vi "testChangeImageBrightness.vi"() -> ()   [LabVIEW 2011, in "run.lvlib"]
uses:
  run.lvlib
  <vilib>/vision/NI_Vision_Development_Module.lvlib
panel:
  out "Maximal Value":sgl
  out "Image Information String":string
  out "Image":T1(plugin-control)
  out "element 2":u32
  in  "stop":bool
  in  "max":dbl(slide) scale=0.0..1604.0
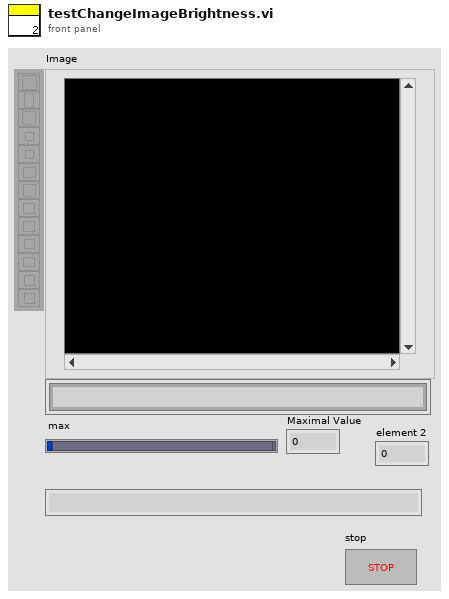
[diagram p1: front panel]
types:
  T1 = typedef "IMAQ Image.ctl" = refnum<image>
  T2 = typedef "Image Type" = u32
  T3 = cluster{"histogram":u32[], "Minimal Value":sgl, "Maximal Value":sgl, "Starting Value":sgl, "Interval Width":sgl, "Mean Value":sgl, "Standard  Variation":sgl, "Area (pixels)":i32}
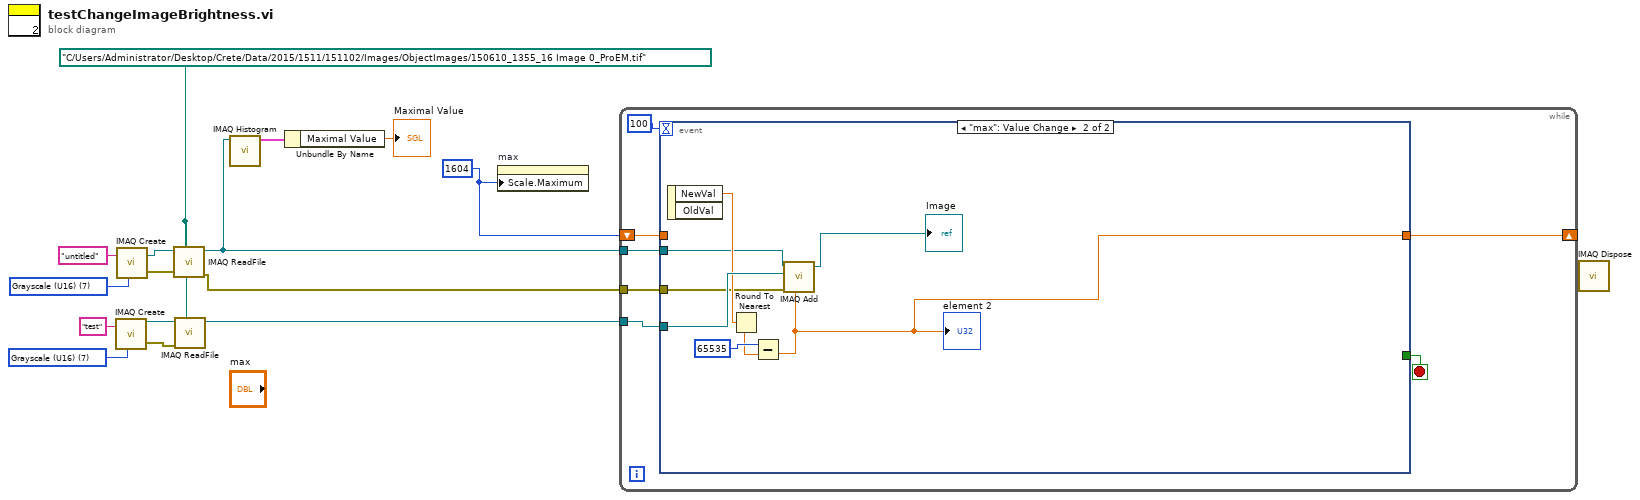
[diagram p0: block diagram]
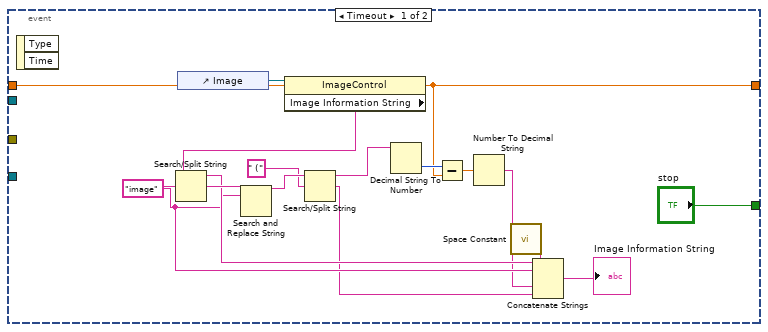
[diagram p2: hidden frame]
diagram:
  w5 = 1604
  w10 = T2 7 items=["Grayscale (U8)", "Grayscale (I16)", "Grayscale (SGL)", "Complex (CSG)", "RGB (U32)", "HSL (U32)", "RGB (U64)", "Grayscale (U16)"] ("Image Type")
  w12 = T2 7 items=["Grayscale (U8)", "Grayscale (I16)", "Grayscale (SGL)", "Complex (CSG)", "RGB (U32)", "HSL (U32)", "RGB (U64)", "Grayscale (U16)"] ("Image Type")
  w7 = path "C:/Users/Administrator/Desktop/Crete/Data/2015/1511/151102/Images/ObjectImages/150610_1355_16 Image 0_ProEM.tif"
  n1 = call "IMAQ Create"("Image Name"="test", "Image Type"=w10) -> ("New Image"=w9:T1, "error out"=w8:errorcluster)  [unwired: 3 in]
  n2 = call "IMAQ Create"("Image Name"="untitled", "Image Type"=w12) -> ("New Image"=w14:T1, "error out"=w15:errorcluster)  [unwired: 3 in]
  n3 = call "IMAQ ReadFile"("File Path"=w7, "error in (no error)"=w15, "Image"=w14) -> ("error out"=w4:errorcluster, "Image Out"=w3:T1)  [unwired: 4 in, 3 out]
  n4 = call "IMAQ ReadFile"("File Path"=w7, "error in (no error)"=w8, "Image"=w9) -> ("Image Out"=w6:T1)  [unwired: 4 in, 4 out]
  n5 = call "IMAQ Histogram"("Image"=w3) -> ("Histogram Report"=w2:T3)  [unwired: 9 in, 1 out]
  n6 = Unbundle By Name(w2) -> ("Maximal Value"=→"Maximal Value":sgl)
  n7 = property on="max" class="Slide (strict)"("Scale.Maximum"=w5) -> ()  [unwired: 2 in, 2 out]
  n8 = while {
    tunnel: w6 -> [w20]
    shift-right: [w19] -> _
    shift-left: w5 -> [w18]
    tunnel: w3 -> [w17]
    tunnel: w4 -> [w16]
    stop <- w22 stop-if-true
    n9 = event shown="[1] \"max\": Value Change" {
      selector: _ -> [_ _]
      dyn-events: _ -> [_ _]
      timeout: 100 -> [_ _]
      tunnel: ["stop" _] -> w22
      tunnel: w20 -> [_ w46]
      tunnel: [w25 w42] -> w19
      tunnel: w18 -> [w25 _]
      tunnel: w17 -> [_ w40]
      tunnel: w16 -> [_ w39]
      event Timeout {
        w29 = "image"
        n10 = event-data() -> ()  [unwired: 1 in, 2 out]
        n11 = control-ref of="Image"() -> (w37:refnum<vi>)
        n12 = property class="ImageControl"(reference=w37) -> ("Image Information String"=w36:string)  [unwired: 1 in, 2 out]
        n13 = Search/Split String(string=w36, search string/char (-)=w29) -> (substring before match=w30:string, match + rest of string=w35:string)  [unwired: 1 in, 1 out]
        n14 = Search and Replace String(input string=w35, search string=w29) -> (result string=w34:string)  [unwired: 6 in, 3 out]
        n15 = Search/Split String(string=w34, search string/char (-)=" (") -> (substring before match=w32:string, match + rest of string=w28:string)  [unwired: 1 in, 1 out]
        n16 = Decimal String To Number(string=w32) -> (number=w26:i32)  [unwired: 2 in, 1 out]
        n17 = Subtract(x=w26, y=w25) -> (x-y=w31:dbl)
        n18 = Number To Decimal String(number=w31) -> (decimal integer string=w24:string)  [unwired: 1 in]
        n19 = call <vilib>:"Space Constant.vi"() -> ("String"=w23:string)
        n20 = Concatenate Strings(w30, w29, w23, w24, w28) -> (→"Image Information String":string)
      }
      event "max": Value Change {
        n21 = event-data() -> ("NewVal"=w43:dbl)  [unwired: 1 in, 1 out]
        n22 = Round To Nearest(number=w43) -> (nearest integer value=w41:dbl)
        n23 = Subtract(x=65535, y=w41) -> (x-y=w42:dbl)
        "element 2" <- w42
        n24 = call "IMAQ Add"("Image Src A"=w40, "Constant"=w42, "Image Dst"=w46, "error in (no error)"=w39) -> ("Image Dst Out"=→"Image":T1)  [unwired: 3 in, 1 out]
      }
    }
  }
  n25 = call "IMAQ Dispose"() -> ()  [unwired: 6 in, 1 out]
